vi "PathPlanner_Path_GetCurveRadiusAtPoint.vi"(9 "Points":T1[](array[typedef]) {"HolonomicRotation"."SIN" format="%13.4f"; "HolonomicRotation"."COS" format="%13.4f"; "HolonomicRotation"."VALUE" format="%13.4f"; "Position"."Y" format="%14.3f"; "Position"."X" format="%14.3f"}, 11 "Index":i32) -> (3 "Radius":dbl)   [LabVIEW 2019, in "PathPlanner24.lvlib"]
doc: "Create a path f\nInputs:\n - \nOutputs:\n - PathPlanner Path -- The generated path"
uses:
  PathPlanner24.lvlib
  TypeDef/PathPlannerPathPoint.ctl
  <vilib>/Rock Robotics/WPI/ThirdParty/JAS_Junk/TrajLib/TypeDef/TRANSLATION2D.ctl
  <vilib>/Rock Robotics/WPI/ThirdParty/JAS_Junk/TrajLib/TypeDef/ROTATION2D.ctl
  TypeDef/PathPlannerPathConstraints.ctl
  <vilib>/Rock Robotics/WPI/ThirdParty/JAS_Junk/TrajLib/Translation2d_GetDistance.vi
  <vilib>/Rock Robotics/WPI/ThirdParty/JAS_Junk/TrajLib/Translation2d_Minus.vi
  <vilib>/Rock Robotics/WPI/ThirdParty/JAS_Junk/TrajLib/Translation2d_GetXY.vi
  <vilib>/Rock Robotics/WPI/ThirdParty/JAS_Junk/TrajLib/Util_CalcDist.vi
  <vilib>/Rock Robotics/WPI/ThirdParty/JAS_Junk/TrajLib/Translation2d_Create.vi
  <vilib>/Rock Robotics/WPI/ThirdParty/JAS_Junk/TrajLib/Trajectory_Library.lvlib
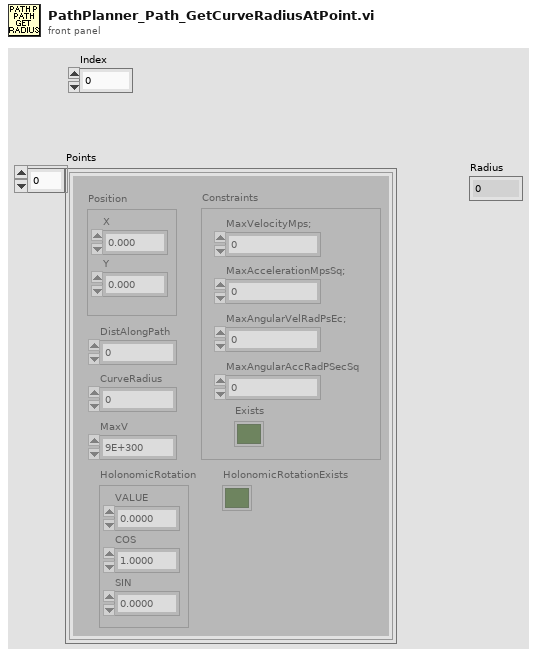
[diagram p1: front panel]
types:
  T1 = typedef "PathPlanner24.lvlib/PathPlannerPathPoint.ctl" = cluster{"Position":T2, "HolonomicRotation":T3, "DistAlongPath":dbl, "CurveRadius":dbl, "MaxV":dbl, "Constraints":T4, "HolonomicRotationExists":bool}
  T2 = typedef "Trajectory_Library.lvlib/TRANSLATION2D.ctl" = cluster{"X":dbl, "Y":dbl}
  T3 = typedef "Trajectory_Library.lvlib/ROTATION2D.ctl" = cluster{"VALUE":dbl, "COS":dbl, "SIN":dbl}
  T4 = typedef "PathPlanner24.lvlib/PathPlannerPathConstraints.ctl" = cluster{"MaxVelocityMps;":dbl, "MaxAccelerationMpsSq;":dbl, "MaxAngularVelRadPsEc;":dbl, "MaxAngularAccRadPSecSq":dbl, "Exists":bool}
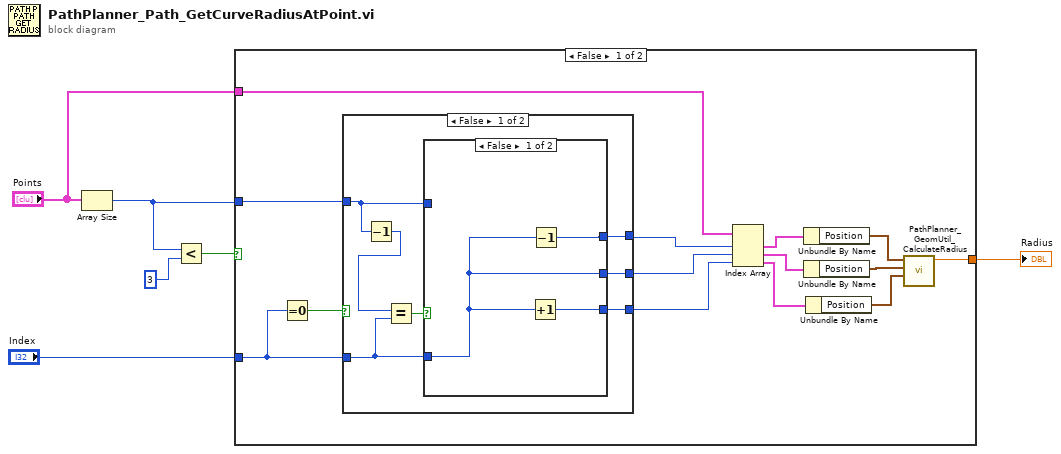
[diagram p0: block diagram]
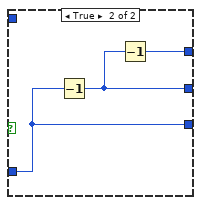
[diagram p2: hidden frame]
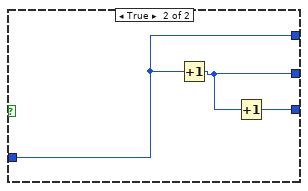
[diagram p3: hidden frame]
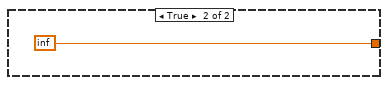
[diagram p4: hidden frame]
diagram:
  n1 = Array Size(array="Points") -> (size(s)=w3:i32)
  n2 = Less?(x=w3, y=3) -> (x < y?=w5:bool)
  n3 = case shown="False" w5 {
    tunnel: [w19 inf] -> w4
    tunnel: w3 -> [w7 _]
    tunnel: "Points" -> [w17 _]
    tunnel: "Index" -> [w18 _]
    frame False {
      n4 = Equal To 0?(x=w18) -> (x = 0?=w20:bool)
      n5 = case shown="False" w20 {
        tunnel: w18 -> [w21 w34]
        tunnel: [w23 w36] -> w16
        tunnel: [w25 w35] -> w15
        tunnel: [w22 w34] -> w14
        tunnel: w7 -> [w24 _]
        frame False {
          n6 = Decrement(x=w24) -> (x-1=w26:i32)
          n7 = Equal?(x=w26, y=w21) -> (x = y?=w27:bool)
          n8 = case shown="False" w27 {
            tunnel: [w30 w31] -> w25
            tunnel: w24 -> [_ _]
            tunnel: [w28 w33] -> w23
            tunnel: [w29 w32] -> w22
            tunnel: w21 -> [w28 w31]
            frame False {
              n9 = Increment(x=w28) -> (x+1=w30:i32)
              n10 = Decrement(x=w28) -> (x-1=w29:i32)
            }
            frame True {
              n11 = Decrement(x=w31) -> (x-1=w33:i32)
              n12 = Decrement(x=w33) -> (x-1=w32:i32)
            }
          }
        }
        frame True {
          n13 = Increment(x=w34) -> (x+1=w36:i32)
          n14 = Increment(x=w36) -> (x+1=w35:i32)
        }
      }
      n15 = Index Array(array=w17, index #1=w14, index #2=w16, index #3=w15) -> (element #1=w13:T1, element #2=w12:T1, element #3=w11:T1)
      n16 = Unbundle By Name(w13) -> ("Position"=w10:T2)
      n17 = Unbundle By Name(w12) -> ("Position"=w9:T2)
      n18 = Unbundle By Name(w11) -> ("Position"=w8:T2)
      n19 = call "PathPlanner_GeomUtil_CalculateRadius.vi"("C"=w8, "B"=w9, "A"=w10) -> ("Radius"=w19:dbl)  [unwired: 8 in]
    }
    frame True {
    }
  }
  "Radius" <- w4
